vi "specrogram.vi"(8 "end of file":bool, 9 "Fs":dbl, 10 "fft size":i32, 11 "Array in":cdb[](array[numeric])) -> (3 "specrogram":T1)   [LabVIEW 2021]
uses:
  <vilib>/Analysis/1siggen.llb/Ramp Pattern by Delta.vi
  <vilib>/measure/maspectr.llb/FFT Power Spectrum and PSD for 1 Chan (CDB).vi
  <vilib>/measure/NI_MAPro.lvlib
  <vilib>/Analysis/NI_AALBase.lvlib
  specrogram_and_param.ctl
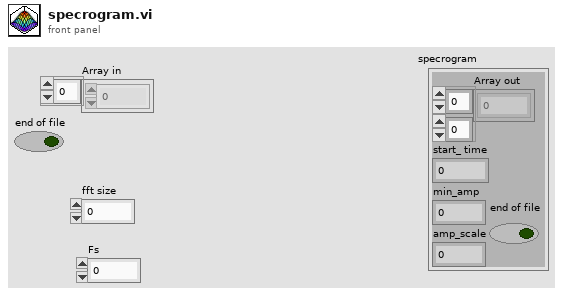
[diagram p1: front panel]
types:
  T1 = typedef "specrogram_and_param.ctl" = cluster{"Array out":sgl[][], "start_ time":dbl, "min_amp":dbl, "amp_scale":dbl, "end of file":bool}
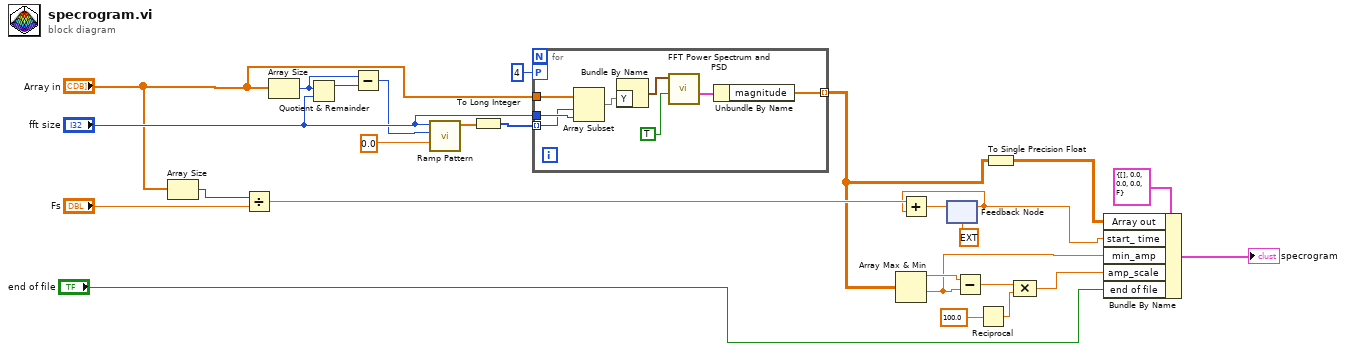
[diagram p0: block diagram]
diagram:
  n1 = Array Size(array="Array in") -> (size(s)=w12:i32)
  n2 = Divide(x=w12, y="Fs") -> (x/y=w11:dbl)
  n3 = Array Size(array="Array in") -> (size(s)=w21:i32)
  n4 = Quotient & Remainder(x=w21, y="fft size") -> (x-y*floor(x/y)=w20:i32)  [unwired: 1 out]
  n5 = Subtract(x=w21, y=w20) -> (x-y=w24:i32)
  n6 = call-poly <vilib>:"Ramp Pattern.vi"("start"=0.0, "end"=w24, "delta"="fft size") -> ("Ramp Pattern"=w23:dbl[])  [unwired: 6 in, 2 out]
  n7 = To Long Integer(number=w23) -> (32bit integer=w22:i32[])
  n8 = for {
    tunnel: [w33] -> w5 mode=indexing
    workers-P: 4 -> [_]
    tunnel: "Array in" -> [w32]
    tunnel: "fft size" -> [w31]
    tunnel: w22 -> [w30] mode=indexing
    n9 = Array Subset(array=w32, index=w30, length=w31) -> (w29:cdb[])
    n10 = Bundle By Name("Y"=w29) -> (w28:waveform(cdb))  [unwired: 1 in]
    n11 = call-poly <vilib>:"FFT Power Spectrum and PSD.vi"("dB On (F)"=TRUE, "time signal"=w28) -> ("Power Spectrum / PSD"=w34:cluster{"f0":dbl, "df":dbl, "magnitude":dbl[]})  [unwired: 6 in, 3 out]
    n12 = Unbundle By Name(w34) -> ("magnitude"=w33:dbl[])
  }
  n13 = Array Max & Min(array=w5) -> (max value=w16:dbl, min value=w7:dbl)  [unwired: 2 out]
  n14 = feedback #1(ext 0.0) -> (w6:ext)
  n15 = Add(x=w11, y=w6) -> (x+y=w9:ext)
  n16 = feedback-in #1(w9) -> ()
  n17 = Subtract(x=w16, y=w7) -> (x-y=w17:dbl)
  n18 = Reciprocal(x=100.0 ("value")) -> (1/x=w18:dbl)
  n19 = To Single Precision Float(number=w5) -> (single precision float=w4:sgl[][])
  n20 = Compound Arithmetic op=MULTIPLY(w17, w18) -> (w8:dbl)
  n21 = Bundle By Name(cluster=T1 {"Array out"=[], "start_ time"=0.0, "min_amp"=0.0, "amp_scale"=0.0, "end of file"=FALSE} ("Cluster"), "Array out"=w4, "start_ time"=w6, "min_amp"=w7, "amp_scale"=w8, "end of file"="end of file") -> (→"specrogram":T1)
